vi "Create Listener.vi"(8 "error in (no error)":errorcluster, 11 "Websocket Server in":refnum<class "Websocket Server.lvclass">) -> (0 "error out":errorcluster, 3 "Websocket Server out":refnum<class "Websocket Server.lvclass">)   [LabVIEW 2020, in "Stream-Websocket.lvlib" / "Websocket Server.lvclass"]
uses:
  Websocket Server.lvclass
  Websocket Server.lvclass/Websocket Server.ctl
  <vilib>/IlluminatedG/lv-stream/Endpoint/Endpoint.lvclass
  <vilib>/IlluminatedG/lv-stream/URI/URI.lvclass
  C:/Program Files (x86)/National Instruments/LabVIEW 2020/vi.lib/IlluminatedG/lv-stream/Endpoint/Endpoint.lvclass
  C:/dev/IlluminatedG/lv-stream-websocket/Stream-Websocket/Websocket Server/Websocket Server.lvclass
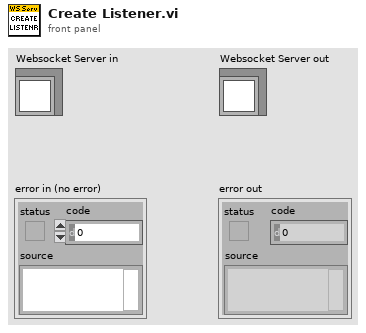
[diagram p1: front panel]
types:
  T1 = typedef "Stream-Websocket.lvlib/Websocket Server.lvclass/Ref Data.ctl" = cluster{"Listener":refnum<k5>, "Clients":refnum<class "Websocket Client.lvclass">[], "Server Loop":bool}
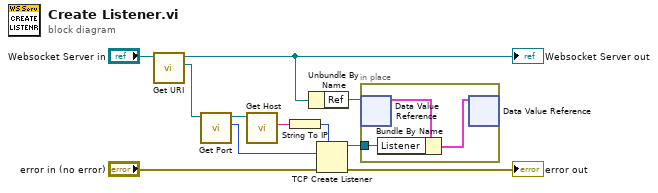
[diagram p0: block diagram]
diagram:
  n1 = call <vilib>:"Get URI.vi"("Endpoint in"="Websocket Server in") -> ("URI"=w10:refnum<class "URI.lvclass">, "Endpoint out"=w3:refnum<class "Websocket Server.lvclass">)  [unwired: 8 in, 1 out]
  "Websocket Server out" <- w3
  n2 = call <vilib>:"Get Port.vi"("URI in"=w10) -> ("Port"=w6:u16, "URI out"=w9:refnum<class "URI.lvclass">)  [unwired: 8 in, 1 out]
  n3 = call <vilib>:"Get Host.vi"("URI in"=w9) -> ("Host"=w8:string)  [unwired: 8 in, 2 out]
  n4 = String To IP(1:w8) -> (0:w7:u32)
  n5 = Unbundle By Name(w3) -> ("Ref"=w4:refnum<data-value>)
  n6 = TCP Create Listener(7:w7, 8:"error in (no error)", 10:w6) -> (0:→"error out":errorcluster, 3:w2:refnum<k5>)  [unwired: 2 in, 1 out]
  n7 = in-place {
    in-place-border: w2 -> [w12]
    n8 = in-place-dvr #1(w4) -> (w14:T1)  [unwired: 1 out]
    n9 = Bundle By Name(cluster=w14, "Listener"=w12) -> (w13:T1)
    n10 = in-place-dvr #1(w13) -> ()  [unwired: 2 out]
  }
